vi "Perform Audio Measurements.vi"(6 "queue":refnum<queue>, 8 "error in":errorcluster, 9 "PCM waveforms":waveform(dbl)[](array[waveform]), 11 "Measurement Configuration":T2={"Analog Source Resource Name"="", "IMD Standard"=0, "Custom Low Frequency"=14000.0, "Custom High frequency"=15000.0, "Custom Amplitude Ratio"=1.0, "Amplitude"=-1.0, "Protocol Source Resource Name"="7821\\PCMi 0", "Input range"=2.825, "Number of Words"=19200, "Clock Rate"=12288000, "Latch Delay"=0.0} {"Custom Amplitude Ratio" format="%.1f"; "Custom High frequency" format="%_2p"; "Custom Low Frequency" format="%#_2p"; "Clock Rate" format="%.4p"}) -> (0 "error out":errorcluster, 3 "Measurement Results":T1)   [LabVIEW 2021, in "audio_intermodulationDistortionMeasurement.lvlib"]
uses:
  audio_intermodulationDistortionMeasurement.lvlib
  <vilib>/addons/_NISVFA/_Shared subVIs/Common/SVL Set dB Reference (1 Ch).vi
  <vilib>/addons/_NISVFA/_Shared subVIs/Common/SVL Set dB Reference (variant).vi
  <vilib>/addons/_NISVFA/_Shared subVIs/Common/svc_Caller VI Returned in Error Source.vi
  <vilib>/addons/Sound and Vibration/svt_Distortion/SVT Intermodulation Distortion (1 Ch).vi
  <vilib>/addons/Sound and Vibration/svt_Distortion/SoundVib_Distortion.lvlib
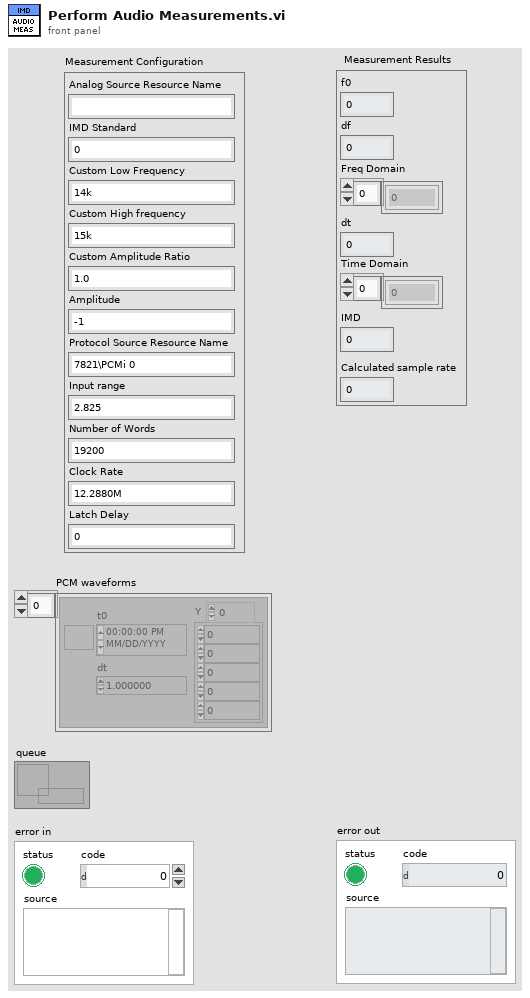
[diagram p1: front panel]
types:
  T1 = cluster{"f0":dbl, "df":dbl, "dt":dbl, "IMD":dbl, "Freq Domain":dbl[], "Time Domain":dbl[], "Calculated sample rate":u32}
  T2 = cluster{"Analog Source Resource Name":string, "IMD Standard":u16, "Custom Low Frequency":dbl, "Custom High frequency":dbl, "Custom Amplitude Ratio":dbl, "Amplitude":dbl, "Protocol Source Resource Name":string, "Input range":dbl, "Number of Words":i32, "Clock Rate":u32, "Latch Delay":dbl}
  T3 = cluster{"IMD type":enum16{"SMPTE/DIN", "CCIF/Twin-Tone"}, "low-frequency tone":dbl, "high-frequency tone":dbl, "amplitude ratio":dbl, "maximum order":i32}
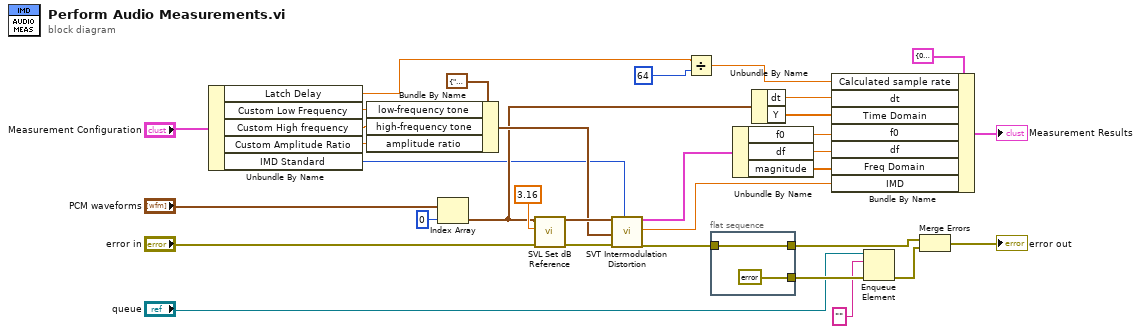
[diagram p0: block diagram]
diagram:
  n1 = Unbundle By Name("Measurement Configuration") -> ("Latch Delay"=w6:dbl, "Custom Low Frequency"=w16:dbl, "Custom High frequency"=w17:dbl, "Custom Amplitude Ratio"=w18:dbl, "IMD Standard"=w7:u16)
  n2 = Bundle By Name(cluster=T3 {"IMD type"=enum."CCIF/Twin-Tone", "low-frequency tone"=14000.0, "high-frequency tone"=15000.0, "amplitude ratio"=1.0, "maximum order"=5} ("custom IMD signal"), "low-frequency tone"=w16, "high-frequency tone"=w17, "amplitude ratio"=w18) -> (w15:T3)
  n3 = Index Array(array="PCM waveforms", index=0) -> (element=w9:waveform(dbl))
  n4 = call-poly <vilib>:"SVL Set dB Reference.vi"("error in (no error)"="error in", "dB reference [EU]"=3.16, "scaled signal in [EU]"=w9) -> ("error out"=w31:errorcluster, "scaled signal out [EU]"=w30:waveform(dbl))  [unwired: 7 in]
  n5 = call-poly <vilib>:"SVT Intermodulation Distortion.vi"("scaled signal [EU]"=w30, "custom IMD signal"=w15, "error in"=w31, "IMD standard"=w7) -> ("magnitude spectrum"=w28:cluster{"f0":dbl, "df":dbl, "magnitude":dbl[]}, "IMD"=w29:dbl, "error out"=w22:errorcluster)  [unwired: 8 in, 5 out]
  n6 = Divide(x=w6, y=u32 64) -> (x/y=w4:dbl)
  n7 = flat-sequence {
    tunnel: w22 -> [w34]
    tunnel: [errorcluster {"status"=FALSE, "code"=0, "source"=""} ("error in (no error)")] -> w23
    tunnel: [w34] -> w13
    frame #0 {
    }
  }
  n8 = Unbundle By Name(w28) -> ("f0"=w27:dbl, "df"=w26:dbl, "magnitude"=w25:dbl[])
  n9 = Unbundle By Name(w9) -> ("dt"=w11:dbl, "Y"=w10:dbl[])
  n10 = Bundle By Name(cluster=T1 {"f0"=0.0, "df"=0.0, "dt"=0.0, "IMD"=0.0, "Freq Domain"=[], "Time Domain"=[], "Calculated sample rate"=0} ("Measurement Results"), "Calculated sample rate"=w4, "dt"=w11, "Time Domain"=w10, "f0"=w27, "df"=w26, "Freq Domain"=w25, "IMD"=w29) -> (→"Measurement Results":T1)
  n11 = Enqueue Element(queue="queue", element="", error in (no error)=w23) -> (error out=w12:errorcluster)  [unwired: 1 in, 2 out]
  n12 = Merge Errors(w13, w12) -> (→"error out":errorcluster)
